vi "KTRL_DECODE.vi"(2 "Etiqueta":string, 4 "Entrada":string) -> (0 "Argumento":string, 1 "Detectado":bool)   [LabVIEW 2017]
panel:
  out "arg":string
  out "cod":string
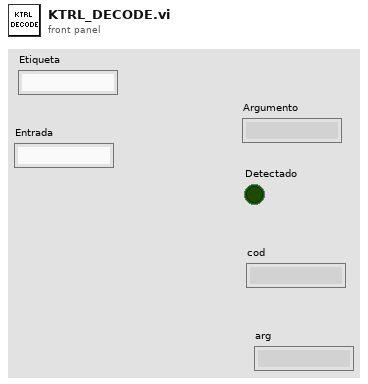
[diagram p1: front panel]
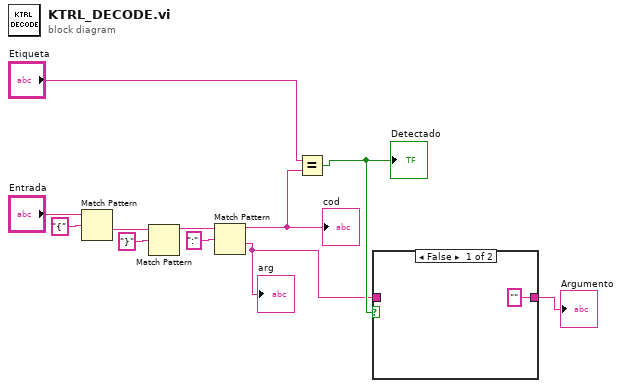
[diagram p0: block diagram]
diagram:
  n1 = Match Pattern(string="Entrada", regular expression="{") -> (after substring=w9:string)  [unwired: 1 in, 3 out]
  n2 = Match Pattern(string=w9, regular expression="}") -> (before substring=w7:string)  [unwired: 1 in, 3 out]
  n3 = Match Pattern(string=w7, regular expression=":") -> (before substring=w4:string, after substring=w1:string)  [unwired: 1 in, 2 out]
  "cod" <- w4
  "arg" <- w1
  n4 = Equal?(x="Etiqueta", y=w4) -> (x = y?=w3:bool)
  "Detectado" <- w3
  n5 = case shown="False" w3 {
    tunnel: ["" ("Entrada") w13] -> w2
    tunnel: w1 -> [_ w13]
    frame False {
    }
    frame True {
    }
  }
  "Argumento" <- w2
